vi "1WIRE_Read_Byte.vi"(8 "error in":errorcluster) -> (0 "error out":errorcluster, 2 "Array":bool[](array[boolean]))   [LabVIEW 2013]
doc: "This VI is created by Vincent Claes for FPDA-1 more information on http://pwo.fpga.be\n\nvincent.claes@xios.be\nclaesvincent@gmail.com\n\nhttp://www.linkedin.com/in/vincentclaes"
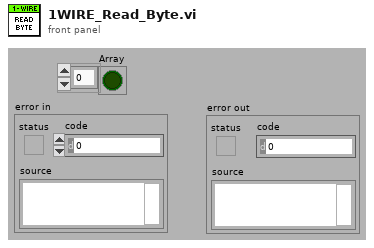
[diagram p1: front panel]
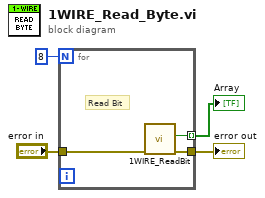
[diagram p0: block diagram]
diagram:
  n1 = for {
    N: 8 -> [_]
    tunnel: [w7] -> w4 mode=indexing
    tunnel: "error in" -> [w6]
    tunnel: [w5] -> w1
    # "Read Bit"
    n2 = call "1WIRE_ReadBit.vi"("error in"=w6) -> ("error out"=w5:errorcluster, "Bit Read"=w7:bool)  [unwired: 9 in]
  }
  "Array" <- w4
  "error out" <- w1
